vi "Pockels modulation control type string to enum.vi"(11 "String":string) -> (3 "Pockels control type":enum16{"NI", "FPGA"}(ring))   [LabVIEW 2017]
uses:
  <vilib>/Utility/error.llb/whitespace.ctl
panel:
  out "string":string
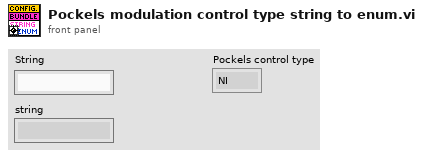
[diagram p1: front panel]
types:
  T1 = typedef "whitespace.ctl" = u16
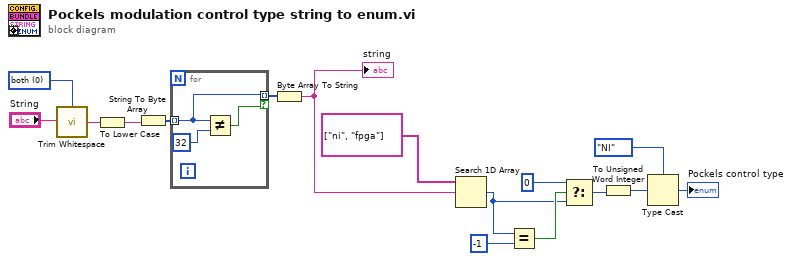
[diagram p0: block diagram]
diagram:
  w13 = T1 0 items=["both", "start of string", "end of string"] ("location (both)")
  n1 = call <vilib>:"Trim Whitespace.vi"("string"="String", "location (both)"=w13) -> ("trimmed string"=w14:string)
  n2 = To Lower Case(string=w14) -> (all lower case string=w16:string)
  n3 = String To Byte Array(string=w16) -> (unsigned byte array=w12:u8[])
  n4 = for {
    tunnel: w12 -> [w18] mode=indexing
    tunnel: [w18] -> w11 mode=indexing if=w17
    n5 = Not Equal?(x=w18, y=u8 32) -> (x != y?=w17:bool)
  }
  n6 = Byte Array To String(unsigned byte array=w11) -> (string=w10:string)
  "string" <- w10
  n7 = Search 1D Array(1D array=string[] ["ni", "fpga"], element=w10) -> (index of element=w5:i32)  [unwired: 1 in]
  n8 = Equal?(x=w5, y=-1) -> (x = y?=w7:bool)
  n9 = Select(t=0, s=w7, f=w5) -> (s? t:f=w2:i32)
  n10 = To Unsigned Word Integer(number=w2) -> (unsigned 16bit integer=w1:u16)
  n11 = Type Cast(type=enum16{"NI", "FPGA"}."NI" ("Laser Power Control HW config.Laser Power Modulation Control 2"), x=w1) -> (*(type *) &x=→"Pockels control type":enum16{"NI", "FPGA"})
